vi "runAScript.vi"(10 "Path":string="\\\\Zeus\\C$\\Documents and Settings\\Administrator\\Desktop\\Crete\\Data\\Scripts\\ScriptRunFolder\\Dipole Trap Script_v2.xml") -> (1 "stoppedByUser":bool, 2 "TimeStamp":string)   [LabVIEW 2009, in "run.lvlib"]
uses:
  run.lvlib
  Viewers/Editors/ExperimentRunner/Events/ExperimentControlEvents.lvclass
  Viewers/ExperimentControl.lvlib
  Events/Event.lvclass
  Tools/Filing/FileNeologist/FileNeologist.lvclass
  Tools/Filing.lvlib
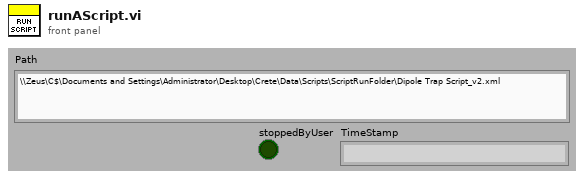
[diagram p1: front panel]
types:
  T1 = enum16{"close", "stopRunning", "runSingleScript", "runExperiment", "runExperimentScript", "Unregistered", "hasStopped"}
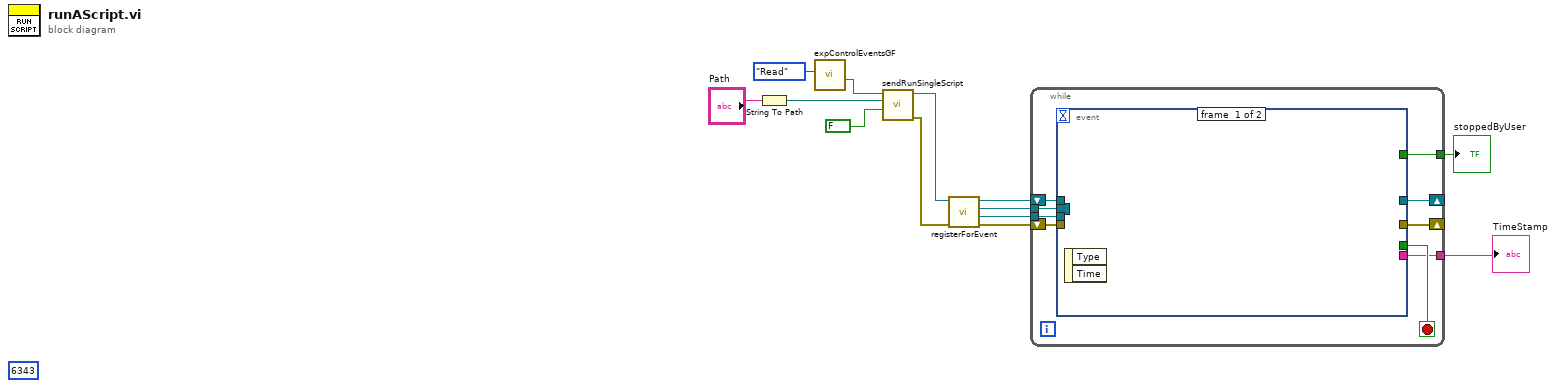
[diagram p0: block diagram]
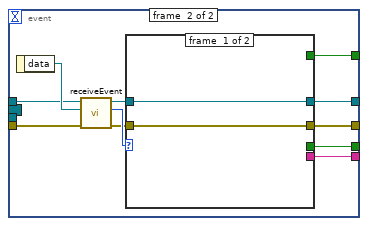
[diagram p2: hidden frame]
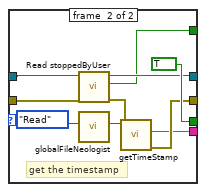
[diagram p3: hidden frame]
diagram:
  (unwired) 6343
  n1 = String To Path(string="Path") -> (path=w11:path)
  n2 = call "expControlEventsGF.vi"("Action"=enum16{"Write", "Read"}."Read") -> ("ExperimentControlEvents"=w10:refnum<class "ExperimentControlEvents.lvclass">)  [unwired: 10 in]
  n3 = call "sendRunSingleScript.vi"("HWLoop"=FALSE, "Path"=w11, "ExperimentControlEvents in"=w10) -> ("error out"=w8:errorcluster, "ExperimentControlEvents out"=w7:refnum<class "ExperimentControlEvents.lvclass">)  [unwired: 7 in]
  n4 = call "registerForEvent.vi"("error in (no error)"=w8, "Event in"=w7) -> ("error out"=w3:errorcluster, "Event"=w5:refnum<user-event>, "Event Registration Refnum"=w6:refnum<event-registration>, "Event out"=w4:refnum<class "ExperimentControlEvents.lvclass">)  [unwired: 6 in]
  n5 = while {
    tunnel: w6 -> [w22]
    tunnel: w5 -> [w21]
    shift-right: [w18] -> _
    shift-left: w4 -> [w20]
    shift-right: [w17] -> _
    shift-left: w3 -> [w19]
    tunnel: [w15] -> w2
    tunnel: [w14] -> w1
    stop <- w16 stop-if-true
    n6 = event shown="[1] <Event>: User Event" {
      selector: w22 -> [_ _]
      dyn-events: _ -> [_ _]
      timeout: _ -> [_ _]
      tunnel: w21 -> [_ _]
      tunnel: w20 -> [_ w32]
      tunnel: w19 -> [_ w31]
      tunnel: [_ w27] -> w18
      tunnel: [_ w28] -> w17
      tunnel: [_ w25] -> w16
      tunnel: [_ w24] -> w15
      tunnel: [_ w23] -> w14
      event #0 {
        n7 = event-data() -> ()  [unwired: 1 in, 2 out]
      }
      event #1 {
        n8 = event-data() -> ("data"=w33:refnum<class>)  [unwired: 1 in]
        n9 = call "receiveEvent.vi"("error in (no error)"=w31, "data"=w33, "ExperimentControlEvents in"=w32) -> ("error out"=w29:errorcluster, "Enum"=w30:T1, "ExperimentControlEvents out"=w26:refnum<class "ExperimentControlEvents.lvclass">)  [unwired: 6 in]
        n10 = case shown="\"hasStopped\"" w30 {
          tunnel: w29 -> [w34 w39]
          tunnel: [w34 w42] -> w28
          tunnel: [w35 w37] -> w27
          tunnel: w26 -> [w35 w40]
          tunnel: [_ TRUE] -> w25
          tunnel: [_ w41] -> w24
          tunnel: [_ w36] -> w23
          frame #0 {
          }
          frame #1 {
            # "get the timestamp"
            n11 = call "Read stoppedByUser.vi"("error in (no error)"=w39, "ExperimentControlEvents in"=w40) -> ("error out"=w38:errorcluster, "stoppedByUser"=w36:bool, "ExperimentControlEvents out"=w37:refnum<class "ExperimentControlEvents.lvclass">)  [unwired: 7 in]
            n12 = call "globalFileNeologist.vi"("Action"=enum16{"Write", "Read"}."Read") -> ("FileNeologist out"=w43:refnum<class "FileNeologist.lvclass">)  [unwired: 10 in]
            n13 = call "getTimeStamp.vi"("error in (no error)"=w38, "FileNeologist in"=w43) -> ("error out"=w42:errorcluster, "TimeStamp"=w41:string)  [unwired: 7 in, 1 out]
          }
        }
      }
    }
  }
  "TimeStamp" <- w2
  "stoppedByUser" <- w1
